vi "format_data.vi"(11 "String":string) -> (3 "Array":dbl[](array[numeric]))   [LabVIEW 2015, in "IMU Custom Device.lvlib"]
uses:
  IMU Custom Device.lvlib
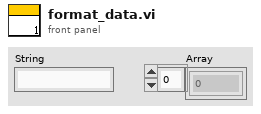
[diagram p1: front panel]
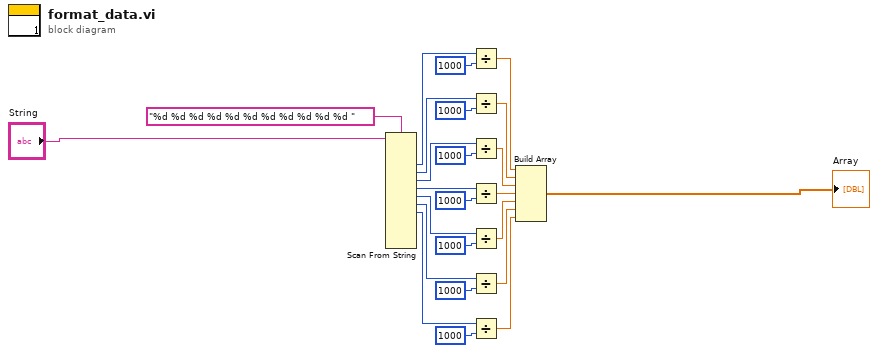
[diagram p0: block diagram]
diagram:
  n1 = Scan From String(format string="%d %d %d %d %d %d %d %d %d %d %d ", input string="String") -> (output 1=w20:i32, output 2=w17:i32, output 3=w16:i32, output 4=w14:i32, output 5=w10:i32, output 6=w9:i32, output 7=w8:i32)  [unwired: 17 in, 3 out]
  n2 = Divide(x=w20, y=1000) -> (x/y=w7:dbl)
  n3 = Divide(x=w17, y=1000) -> (x/y=w6:dbl)
  n4 = Divide(x=w16, y=1000) -> (x/y=w5:dbl)
  n5 = Divide(x=w14, y=1000) -> (x/y=w4:dbl)
  n6 = Divide(x=w10, y=1000) -> (x/y=w3:dbl)
  n7 = Divide(x=w9, y=1000) -> (x/y=w2:dbl)
  n8 = Divide(x=w8, y=1000) -> (x/y=w1:dbl)
  n9 = Build Array(w7, w6, w5, w4, w3, w2, w1) -> (→"Array":dbl[])
